vi "createModule.vi"(8 "error in (no error)":errorcluster, 9 "moduleContentsString":string, 10 "moduleName":string, 11 "IDLFile in":refnum<class "IDLFile.lvclass">) -> (0 "error out":errorcluster, 3 "IDLFile out":refnum<class "IDLFile.lvclass">)   [LabVIEW 2016, in "IDLFile.lvclass"]
uses:
  IDLFile.lvclass
  IDLFile.lvclass/IDLFile.ctl
  Module/Module.lvclass/Module.ctl
  Module/Module.lvclass
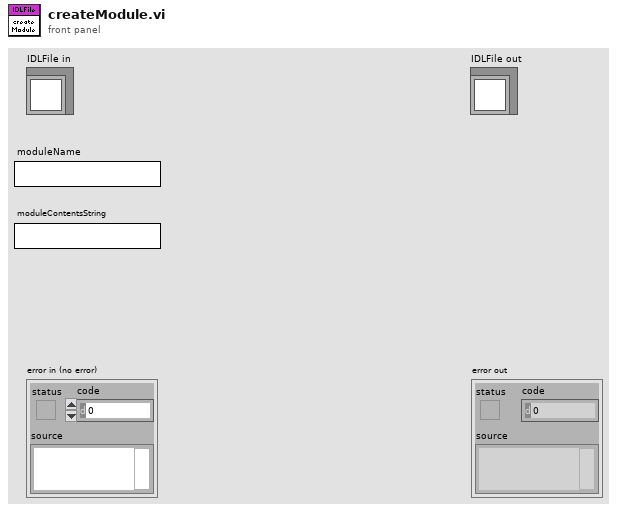
[diagram p1: front panel]
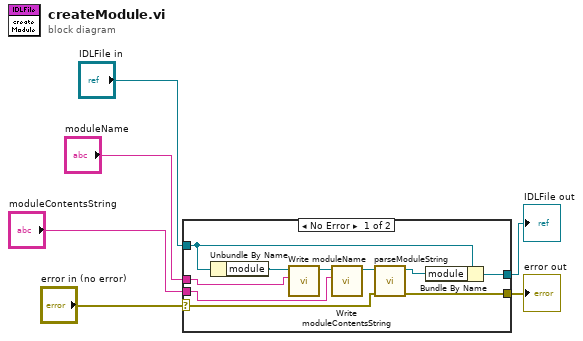
[diagram p0: block diagram]
diagram:
  n1 = case shown="No Error" "error in (no error)" {
    selector: "error in (no error)" -> [w8 w18]
    tunnel: [w7 w18] -> w5
    tunnel: [w11 w17] -> w3
    tunnel: "IDLFile in" -> [w12 w17]
    tunnel: "moduleName" -> [w15 _]
    tunnel: "moduleContentsString" -> [w13 _]
    frame No Error {
      n2 = Unbundle By Name(w12) -> ("module"=w16:refnum<class "Module.lvclass">)
      n3 = call "Write moduleName.vi"("moduleName"=w15, "Module in"=w16) -> ("Module out"=w14:refnum<class "Module.lvclass">)  [unwired: 9 in]
      n4 = call "Write moduleContentsString.vi"("moduleContentsString"=w13, "Module in"=w14) -> ("Module out"=w10:refnum<class "Module.lvclass">)  [unwired: 9 in]
      n5 = call "parseModuleString.vi"("error in (no error)"=w8, "Module in"=w10) -> ("error out"=w7:errorcluster, "Module out"=w9:refnum<class "Module.lvclass">)  [unwired: 8 in]
      n6 = Bundle By Name(cluster=w12, "module"=w9) -> (w11:refnum<class "IDLFile.lvclass">)
    }
    frame Error {
    }
  }
  "error out" <- w5
  "IDLFile out" <- w3
